vi "Lakeshore 218 Rd Wr Settings.vi"(8 "error in (no error)":errorcluster, 10 "Write? (F:Read)":bool, 11 "LS 218 Settings":T1={"Port"="Lakeshore218", "Channel Names"=["Unused 1", "Unused 2", "Unused 3", "Unused 4", "Unused 5", "Unused 6", "Unused 7", "Unused 8"], "Ch Enable"=[FALSE, FALSE, FALSE, FALSE, FALSE, FALSE, FALSE, FALSE]}) -> (0 "error out":errorcluster, 3 "LS 218 Settings":T1={"Port"="Lakeshore218", "Channel Names"=[], "Ch Enable"=[]})   [LabVIEW 2024, in "Lakeshore 218.lvclass"]
uses:
  Lakeshore 218.lvclass
  Lakeshore 218 cluster Settings.ctl
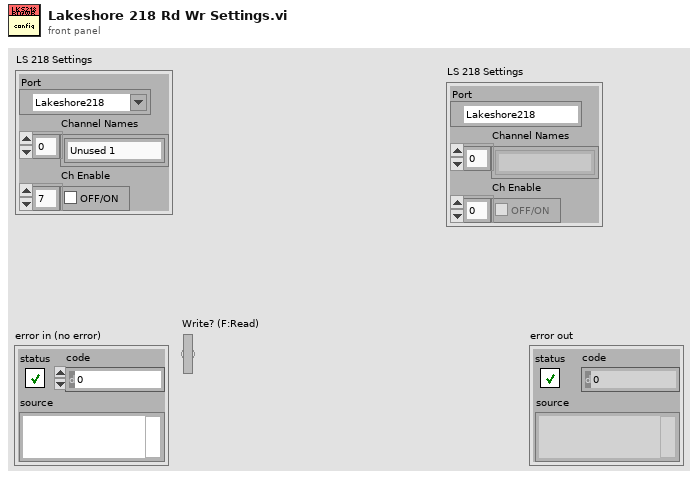
[diagram p1: front panel]
types:
  T1 = typedef "Lakeshore 218.lvclass/Lakeshore 218 cluster Settings.ctl" = cluster{"Port":refnum<visa-resource-name>, "Channel Names":string[], "Ch Enable":bool[]}
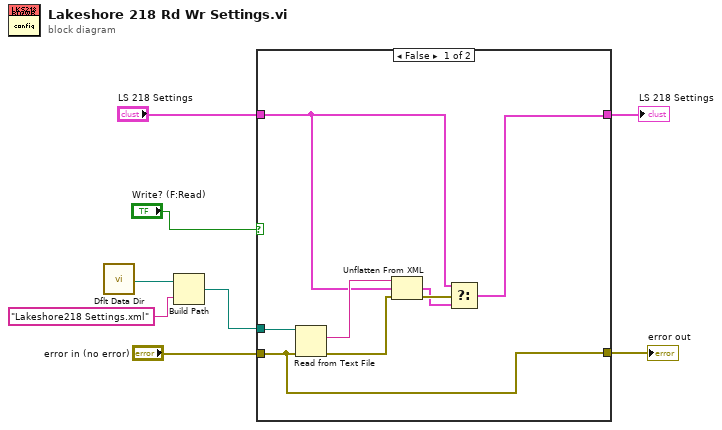
[diagram p0: block diagram]
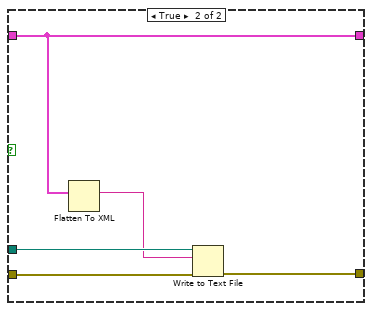
[diagram p2: hidden frame]
diagram:
  n1 = call <vilib>:"Dflt Data Dir.vi"() -> ("App:Default Data Directory"=w5:path)
  n2 = Build Path(base path=w5, name or relative path="Lakeshore218 Settings.xml") -> (appended path=w4:path)
  n3 = case shown="False" "Write? (F:Read)" {
    tunnel: "error in (no error)" -> [w9 w21]
    tunnel: "LS 218 Settings" -> [w12 w17]
    tunnel: w4 -> [w16 w20]
    tunnel: [w9 w18] -> w3
    tunnel: [w10 w17] -> w2
    frame False {
      n4 = Read from Text File(file (use dialog)=w16, error in=w9) -> (text=w15:string, error out=w14:errorcluster)  [unwired: 2 in, 2 out]
      n5 = Unflatten From XML(xml string=w15, type=w12, error in (no error)=w14) -> (value=w11:T1, error out=w13:errorcluster)
      n6 = Select(t=w12, s=w13, f=w11) -> (s? t:f=w10:T1)
    }
    frame True {
      n7 = Flatten To XML(6:w17) -> (2:w19:string)
      n8 = Write to Text File(file (use dialog)=w20, text=w19, error in=w21) -> (error out=w18:errorcluster)  [unwired: 1 in, 2 out]
    }
  }
  "error out" <- w3
  "LS 218 Settings" <- w2
